vi "SetMotors.vi"() -> ()   [LabVIEW 2018]
uses:
  <vilib>/Studica/Studica Toolkit/Background/Mxp Selection.ctl
panel:
  in  "1":dbl(slide)=-0.0 scale=-1.0..1.0
  in  "2":dbl(slide)=-0.0 scale=-1.0..1.0
  in  "3":dbl(slide)=-0.0 scale=-1.0..1.0
  in  "4":dbl(slide) scale=-1.0..1.0
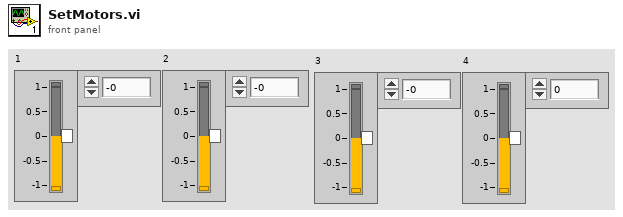
[diagram p1: front panel]
types:
  T1 = typedef "Mxp Selection.ctl" = enum16{"MXP A", "MXP B"}
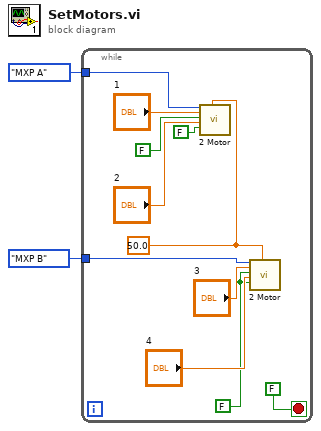
[diagram p0: block diagram]
diagram:
  n1 = while {
    tunnel: Mxp_Selection."MXP A" ("Mxp Side") -> [w13]
    tunnel: Mxp_Selection."MXP B" ("Mxp Side") -> [w12]
    stop <- FALSE stop-if-true
    w7 = 50.0 ("Frequency [Hz]")
    w3 = FALSE ("Invert M0")
    n2 = call <vilib>:"2 Motor.vi"("Mxp Side"=w13, "Speed M0"="1", "Invert M0"=FALSE, "Speed M1"="2", "Invert M1"=FALSE ("Invert M0"), "Frequency [Hz]"=w7) -> ()  [unwired: 13 in, 1 out]
    n3 = call <vilib>:"2 Motor.vi"("Mxp Side"=w12, "Speed M0"="3", "Invert M0"=w3, "Speed M1"="4", "Invert M1"=w3, "Frequency [Hz]"=w7) -> ()  [unwired: 13 in, 1 out]
  }
